vi "DO Write Line.vi"(7 "Value":u16, 8 "error in (no error)":errorcluster caption="错误输入（无错误）", 9 "Line":u16, 10 "Port":u16, 11 "CardNumber":u16) -> (0 "error out":errorcluster caption="错误输出", 3 "function return":i16)   [LabVIEW 2017, in "Adlink IO.lvlib"]
doc: "I16 __stdcall DO_WriteLine(U16 CardNumber, U16 Port, U16 Line, U16 Value);"
uses:
  Adlink IO.lvlib
  PCI-Dask.dll
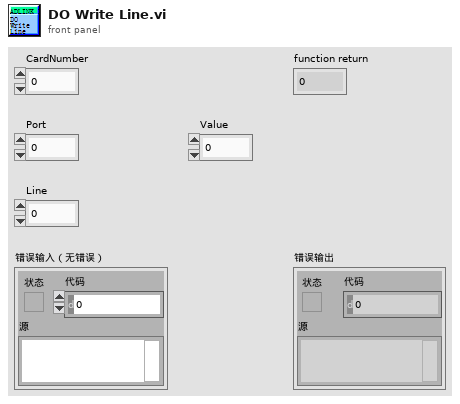
[diagram p1: front panel]
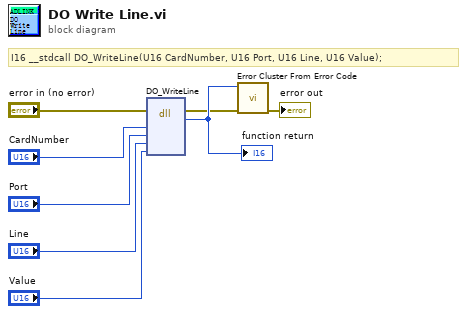
[diagram p0: block diagram]
diagram:
  # "I16 __stdcall DO_WriteLine(U16 CardNumber, U16 Port, U16 Line, U16 Value);"
  n1 = dll-call lib="D:/X682 Camera Calibration Tester Program/HardWare/ADLINK/IO/Adlink IO/PCI-Dask.*" fn="DO_WriteLine"(error in="error in (no error)", "CardNumber"="CardNumber", "Port"="Port", "Line"="Line", "Value"="Value") -> (error out=w2:errorcluster, w8:i16)  [unwired: 6 in, 1 out]
  "function return" <- w8
  n2 = call <vilib>:"Error Cluster From Error Code.vi"("error in (no error)"=w2, "error code (0)"=w8) -> ("error out"=→"error out":errorcluster)  [unwired: 7 in]
